vi "ROI_to_rects.vi"(0 "binning":cluster{"x":u8, "y":u8}={"x"=1, "y"=1}, 1 "ROI":T2) -> (2 "center":cluster{"x":i16, "y":i16}, 3 "rect array":i32[](array[numeric]), 4 "rect":T1, 5 "valid":bool)   [LabVIEW 2010]
uses:
  <userlib>/bias2/subvis/ROI_rect.ctl
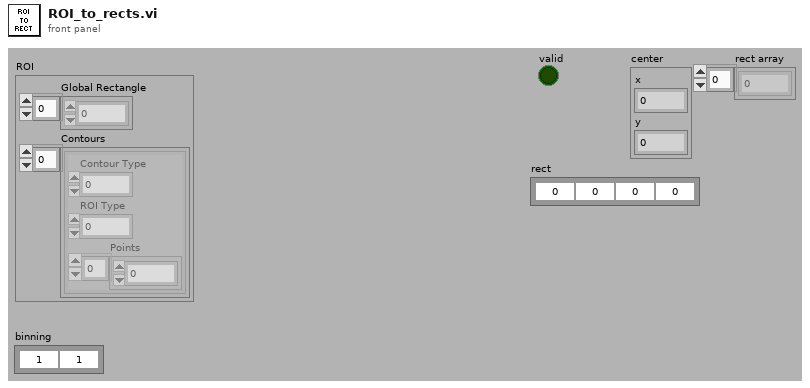
[diagram p1: front panel]
types:
  T1 = typedef "ROI_rect.ctl" = cluster{"left":i32, "top":i32, "right":i32, "bottom":i32}
  T2 = cluster{"Global Rectangle":i32[], "Contours":cluster{"Contour Type":u32, "ROI Type":u32, "Points":i32[]}[]}
  T3 = cluster{"Contour Type":u32, "ROI Type":u32, "Points":i32[]}[]
  T4 = cluster{"[0]":i32, "[1]":i32, "[2]":i32, "[3]":i32}
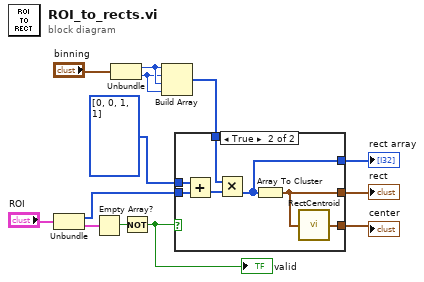
[diagram p0: block diagram]
diagram:
  n1 = Unbundle("ROI") -> ("Global Rectangle"=w9:i32[], "Contours"=w12:T3)
  n2 = Empty Array?(array=w12) -> (empty?=w11:bool)
  n3 = Unbundle("binning") -> ("x"=w3:u8, "y"=w2:u8)
  n4 = Not(x=w11) -> (.not. x?=w10:bool)
  "valid" <- w10
  n5 = Build Array(w3, w2, w3, w2) -> (w1:u8[])
  n6 = case shown="True" w10 {
    tunnel: w9 -> [_ w17]
    tunnel: [_ w19] -> w8
    tunnel: [_ w20] -> w7
    tunnel: [_ w15] -> w6
    tunnel: i32[] [0, 0, 1, 1] ("array") -> [_ w16]
    tunnel: w1 -> [_ w14]
    frame False {
    }
    frame True {
      n7 = Add(x=w16, y=w17) -> (x+y=w18:i32[])
      n8 = Multiply(x=w14, y=w18) -> (x*y=w15:i32[])
      n9 = Array To Cluster(array=w15) -> (cluster=w19:T4)
      n10 = call <vilib>:"RectCentroid.vi"("rect"=w19) -> ("point"=w20:cluster{"x":i16, "y":i16})
    }
  }
  "rect" <- w8
  "center" <- w7
  "rect array" <- w6
